vi "HDF5_LogArray.vi"(8 "error in (no error)":errorcluster, 10 "array of Data":dbl[](array[numeric]), 11 "array of Refs":T1[](array[typedef]) format="%.0x") -> (0 "error out":errorcluster)   [LabVIEW 2018]
uses:
  <vilib>/addons/h5labview2/base/hid_t.ctl
  lib_path_mod_20200519.vi
  <vilib>/addons/h5labview2/base/H5Equery.vi
  <vilib>/addons/h5labview2/dataset/H5Dwrite.llb/H5Dwrite.xnode
  <vilib>/addons/h5labview2/dataset/H5D.lvlib
  <vilib>/addons/h5labview2/space/H5S.lvlib
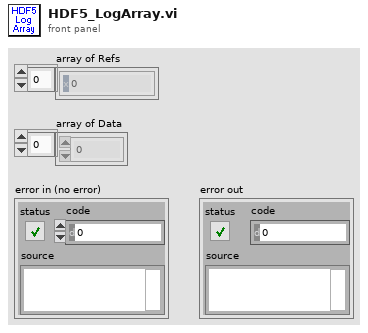
[diagram p1: front panel]
types:
  T1 = typedef "hid_t.ctl" = i32
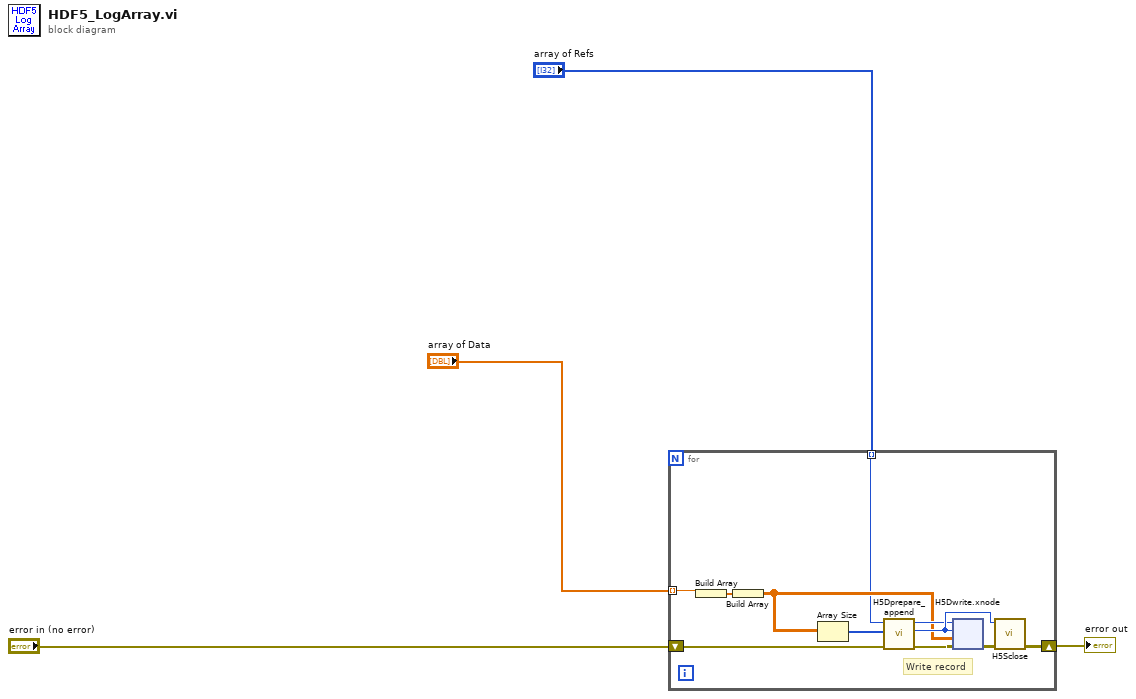
[diagram p0: block diagram]
diagram:
  n1 = for {
    shift-right: [w11] -> w2
    shift-left: "error in (no error)" -> [w7]
    tunnel: "array of Refs" -> [w6] mode=indexing
    tunnel: "array of Data" -> [w5] mode=indexing
    # "Write record"
    n2 = Build Array(w5) -> (w10:dbl[])
    n3 = Build Array(w10) -> (w9:dbl[][])
    n4 = Array Size(array=w9) -> (size(s)=w8:i32[])
    n5 = call <vilib>:"H5Dprepare_append.vi"("error in (no error)"=w7, "append dims"=w8, "dset in"=w6) -> ("error out"=w15:errorcluster, "space out"=w13:T1, "dset out"=w12:T1)  [unwired: 5 in, 1 out]
    n6 = xnode "H5Dwrite.xnode"("error in (no error)"=w15, "data"=w9, "file space"=w13, "ref in"=w12) -> ("error out"=w14:errorcluster)  [unwired: 3 in, 2 out]
    n7 = call <vilib>:"H5Sclose.vi"("error in (no error)"=w14, "space in"=w13) -> ("error out"=w11:errorcluster)  [unwired: 9 in]
  }
  "error out" <- w2
